vi "Get_Default_Install_Path.vi"(8 "error in (no error)":errorcluster, 11 "Installer in":refnum<class "Installer.lvclass">) -> (0 "error out":errorcluster, 2 "default_installPath":string, 3 "Installer out":refnum<class "Installer.lvclass">)   [LabVIEW 2020, in "Installer.lvclass"]
uses:
  <vilib>/AppBuilder/IB_Classes/Installer/Installer.lvclass
  <vilib>/AppBuilder/IB_Classes/Installer/Installer.lvclass/Installer.ctl
  <vilib>/AppBuilder/IB_Classes/Destination/IB_Destination.lvclass
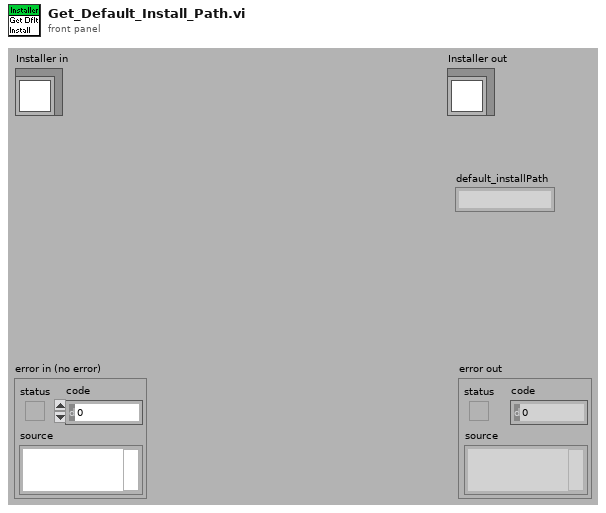
[diagram p1: front panel]
types:
  T1 = typedef "IB_Destination.ctl" = cluster{"name":string, "unlock":bool, "parentTag":string, "destTag":string, "eng_installPath":string}
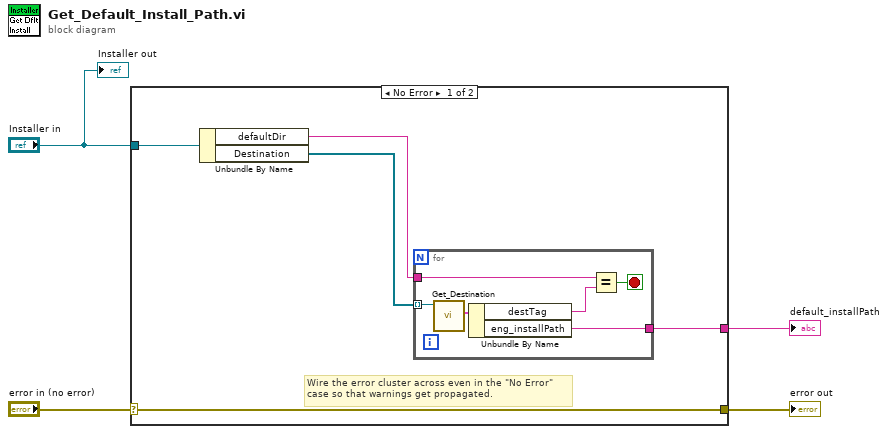
[diagram p0: block diagram]
diagram:
  n1 = case shown="No Error" "error in (no error)" {
    selector: "error in (no error)" -> [w9 w16]
    tunnel: [w9 w16] -> w3
    tunnel: "Installer in" -> [w7 _]
    tunnel: [w5 _] -> w1
    frame No Error {
      # "Wire the error cluster across even in the \"No Error\"\ncase so that warnings get propagated."
      n2 = Unbundle By Name(w7) -> ("defaultDir"=w6:string, "Destination"=w8:refnum<class "IB_Destination.lvclass">[])
      n3 = for {
        tunnel: w8 -> [w15] mode=indexing
        tunnel: w6 -> [w13]
        tunnel: [w10] -> w5
        stop <- w11 stop-if-true
        n4 = call <vilib>:"Get_Destination.vi"("IB_Destination in"=w15) -> ("data"=w14:T1)  [unwired: 1 in, 9 out]
        n5 = Unbundle By Name(w14) -> ("destTag"=w12:string, "eng_installPath"=w10:string)
        n6 = Equal?(x=w13, y=w12) -> (x = y?=w11:bool)
      }
    }
    frame Error {
    }
  }
  "error out" <- w3
  "default_installPath" <- w1
  "Installer out" <- "Installer in"
